vi "Write metadatas.vi"(8 "error in (no error)":errorcluster, 10 "metadatas":cluster{"key":string, "value":string}[](array[cluster]), 11 "data_node in":refnum<class "data_node.lvclass">) -> (0 "error out":errorcluster, 3 "data_node out":refnum<class "data_node.lvclass">)   [LabVIEW 2020, in "data_node.lvclass"]
uses:
  data_node.lvclass
  data_node.lvclass/data_node.ctl
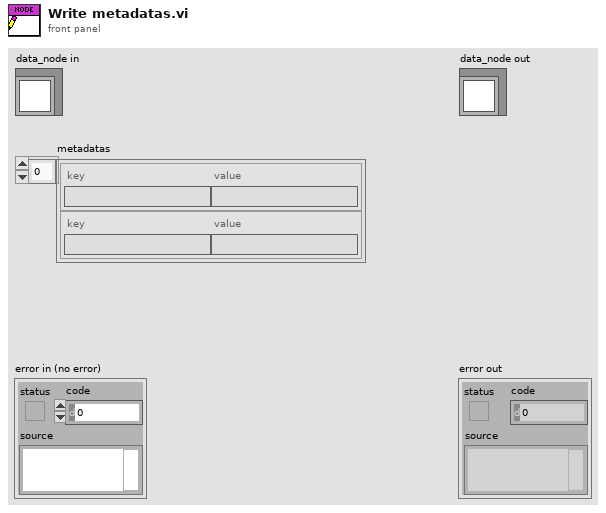
[diagram p1: front panel]
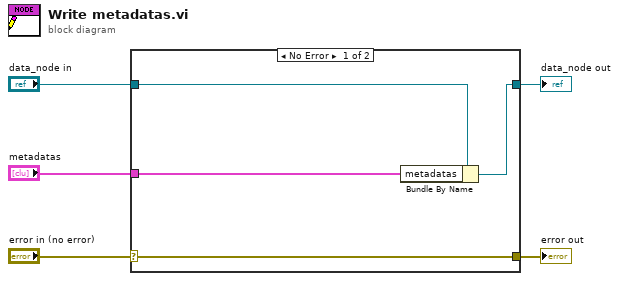
[diagram p0: block diagram]
diagram:
  n1 = case shown="No Error" "error in (no error)" {
    selector: "error in (no error)" -> [w9 w10]
    tunnel: [w9 w10] -> w4
    tunnel: [w7 w11] -> w2
    tunnel: "data_node in" -> [w8 w11]
    tunnel: "metadatas" -> [w6 _]
    frame No Error {
      n2 = Bundle By Name(cluster=w8, "metadatas"=w6) -> (w7:refnum<class "data_node.lvclass">)
    }
    frame Error {
    }
  }
  "error out" <- w4
  "data_node out" <- w2
